vi "IndParamArray.vi"(9 "Step Sizes":dbl[](array[numeric]), 10 "Final Values":dbl[](array[numeric]), 11 "Initial Values":dbl[](array[numeric])) -> (3 "Array":dbl[](array[numeric]))   [LabVIEW 2013]
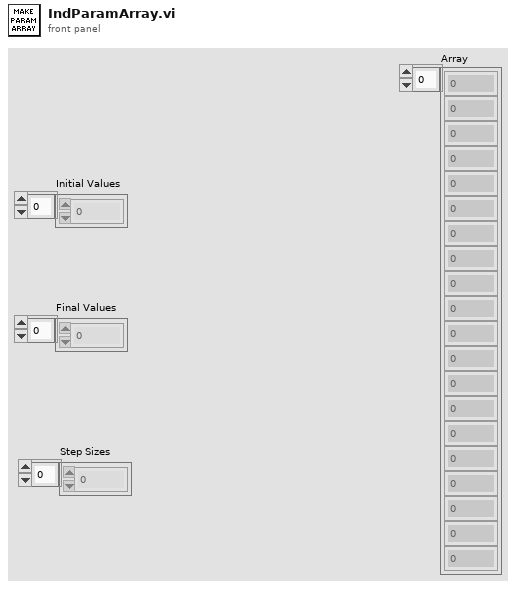
[diagram p1: front panel]
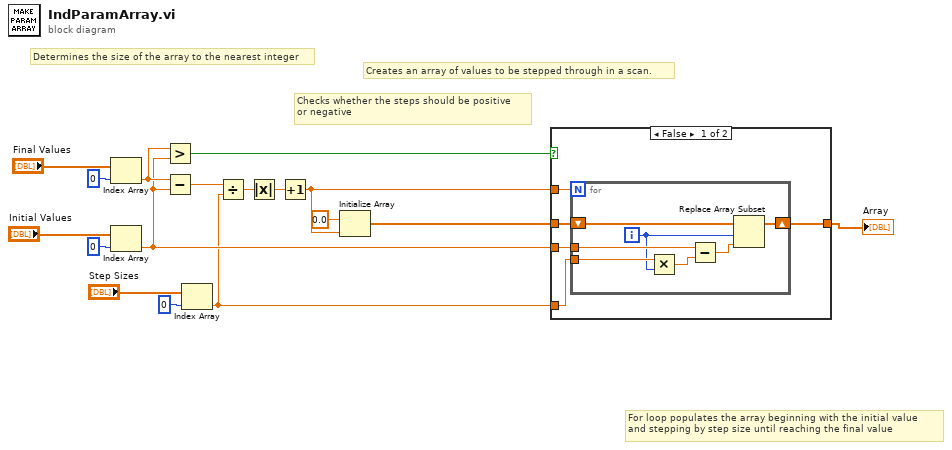
[diagram p0: block diagram]
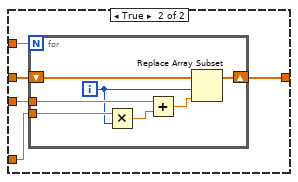
[diagram p2: hidden frame]
diagram:
  # "For loop populates the array beginning with the initial value\nand stepping by step size until reaching the final value"
  # "Determines the size of the array to the nearest integer"
  # "Checks whether the steps should be positive\nor negative"
  # "Creates an array of values to be stepped through in a scan."
  n1 = Index Array(array="Final Values", index=0) -> (element=w3:dbl)
  n2 = Index Array(array="Initial Values", index=0) -> (element=w2:dbl)
  n3 = Greater?(x=w3, y=w2) -> (0:w14:bool)
  n4 = Subtract(x=w3, y=w2) -> (x-y=w17:dbl)
  n5 = Index Array(array="Step Sizes", index=0) -> (element=w1:dbl)
  n6 = Divide(x=w17, y=w1) -> (x/y=w15:dbl)
  n7 = Absolute Value(x=w15) -> (abs(x)=w11:dbl)
  n8 = Increment(x=w11) -> (x+1=w10:dbl)
  n9 = Initialize Array(0.0 ("element"), w10) -> (w13:dbl[])
  n10 = case shown="False" w14 {
    tunnel: w13 -> [w20 w34]
    tunnel: w10 -> [w22 w33]
    tunnel: w1 -> [w19 w32]
    tunnel: w2 -> [w18 w31]
    tunnel: [w21 w30] -> w12
    frame False {
      n11 = for {
        N: w22 -> [_]
        shift-right: [w23] -> w21
        shift-left: w20 -> [w24]
        tunnel: w19 -> [w29]
        tunnel: w18 -> [w28]
        i -> [w26]
        n12 = Multiply(x=w29, y=w26) -> (x*y=w27:dbl)
        n13 = Subtract(x=w28, y=w27) -> (x-y=w25:dbl)
        n14 = Replace Array Subset(array=w24, new element=w25, index=w26) -> (w23:dbl[])
      }
    }
    frame True {
      n15 = for {
        N: w33 -> [_]
        shift-right: [w40] -> w30
        shift-left: w34 -> [w41]
        tunnel: w32 -> [w39]
        tunnel: w31 -> [w38]
        i -> [w35]
        n16 = Multiply(x=w39, y=w35) -> (x*y=w37:dbl)
        n17 = Add(x=w38, y=w37) -> (x+y=w36:dbl)
        n18 = Replace Array Subset(array=w41, new element=w36, index=w35) -> (w40:dbl[])
      }
    }
  }
  "Array" <- w12
